vi "Shooter Immediate_wrapper.vi"() -> ()   [LabVIEW 2025]
uses:
  <vilib>/Rock Robotics/WPI/Framework/Command Status Info.ctl
  <vilib>/Rock Robotics/WPI/Framework/Completion Status.ctl
  <vilib>/Rock Robotics/WPI/Framework/Completion Notifier.ctl
  Implementation/Shooter Operations.ctl
panel:
  out "Command Info Out":T1
  in  "Setpoint":dbl
  in  "Hood Setpoint":dbl
  in  "Operation":T4
  in  "Command Info In":T1
  in  "Description":string
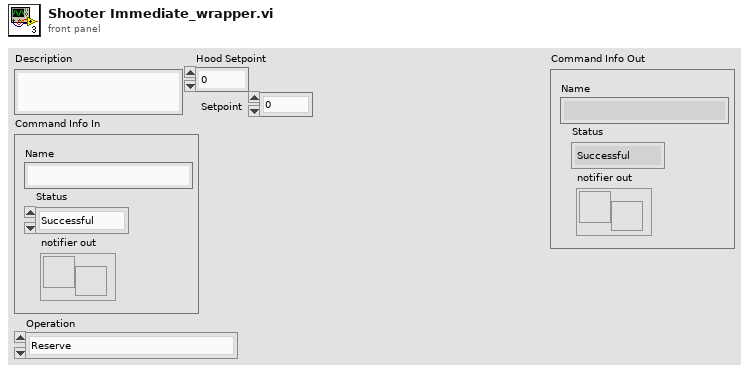
[diagram p1: front panel]
types:
  T1 = typedef "Command Status Info.ctl" = cluster{"Name":string, "Status":T2, "notifier out":T3}
  T2 = typedef "Completion Status.ctl" = enum16{"Successful", "Aborted", "Incomplete"}
  T3 = typedef "Completion Notifier.ctl" = refnum<notifier>
  T4 = typedef "Shooter Operations.ctl" = enum16{"Reserve", "Read Current", "Interpolated Shot", "Hood Manual", "Reset Hood", "Immediate", "Start Shooter"}
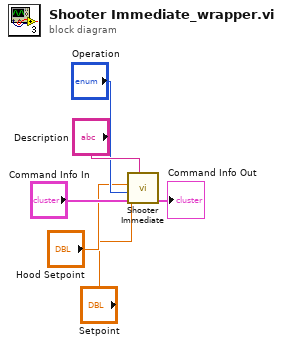
[diagram p0: block diagram]
diagram:
  n1 = call "Shooter Immediate.vi"("Description"="Description", "Command Info In"="Command Info In", "Operation"="Operation", "Hood Setpoint"="Hood Setpoint", "Setpoint"="Setpoint") -> ("Command Info Out"=→"Command Info Out":T1)  [unwired: 6 in]
